vi "newTest.vi"(8 "error in (no error)":errorcluster, 11 "Data in":T1={"Report.lvclass"=refnum, "Norm"="", "last State"=enum."Initialize", "Norm ID"=0, "parameter"=[], "EMTestCWS500N.lvclass"=refnum, "CEG4500.lvclass"=refnum, "Tektronix RSA5106A.lvclass"=refnum, "erfolgreich"=FALSE, "log"="", "Kommentar"="", "Device Enum"=enum."emTestCWS500N", "Test Enum"=enum."HF-Felder", "debug"=FALSE, "tab"=enum."Hauptmenü", "ESD Pistol.lvclass"=refnum, "SubPnl Refnum"=refnum, "TabCtl Refnum"=refnum, "ButtonsEinblenden?"=FALSE}) -> (0 "error out":errorcluster, 2 "abbrechen":bool, 3 "Test out":refnum<class "Test.lvclass">)   [LabVIEW 2013]
uses:
  Main/controls/Data.ctl
  classes/Datastructure/Report/Report.lvclass
  classes/Devices/emTestCWS500N/EMTestCWS500N.lvclass
  classes/Devices/CEG4500/CEG4500.lvclass
  classes/Devices/Tektronix RSA5106A/Tektronix RSA5106A.lvclass
  ESD Pistol.lvclass
  Main/controls/State.ctl
  classes/Devices/DeviceInterface/Devices.ctl
  classes/Tests/TestInterface/Tests.ctl
  Tabs.ctl
  classes/Datastructure/Test/Test.lvclass
  classes/Datastructure/Norm/Norm.lvclass
  classes/Datastructure/Image/img.lvclass
panel:
  in  "Cancel Button":bool
  in  "Tree 2":string(tree)
  out "Norm":string caption="Test"
  in  "OK Button":bool
  in  "Add picture":bool
  in  "Kommentar":string
  in  "Test Name":string
  in  "Parameter":string[][](table)
  in  "number of pictures":i32
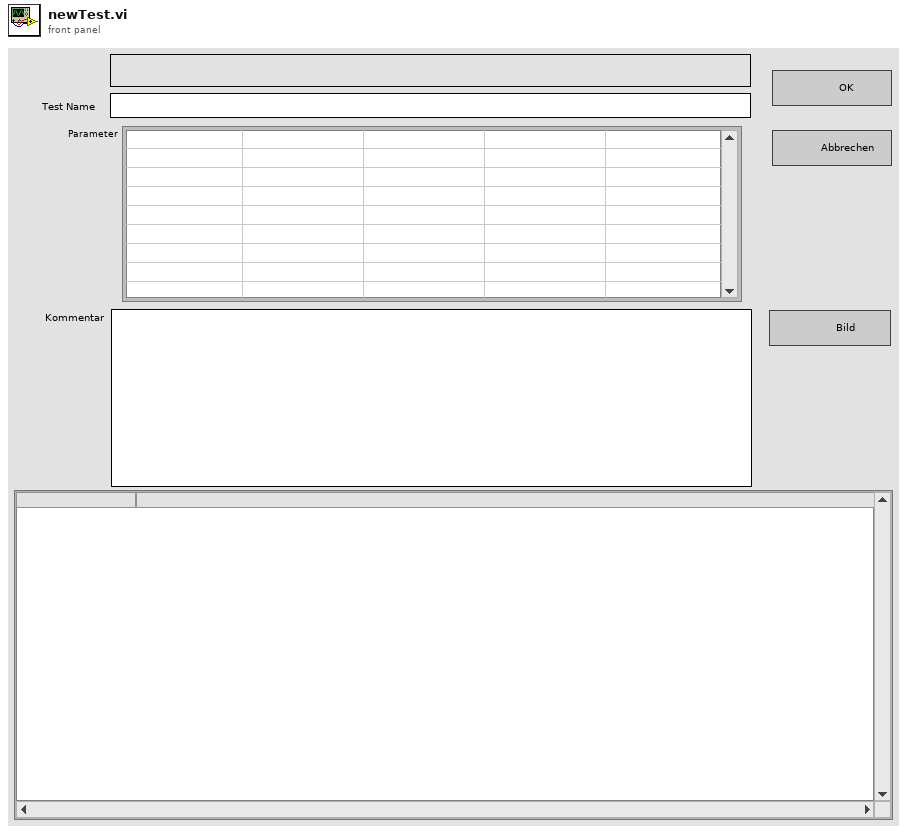
[diagram p1: front panel]
types:
  T1 = typedef "Data.ctl" = cluster{"Report.lvclass":refnum<class "Report.lvclass">, "Norm":string, "last State":T2, "Norm ID":i32, "parameter":string[][], "EMTestCWS500N.lvclass":refnum<class "EMTestCWS500N.lvclass">, "CEG4500.lvclass":refnum<class "CEG4500.lvclass">, "Tektronix RSA5106A.lvclass":refnum<class "Tektronix RSA5106A.lvclass">, "erfolgreich":bool, "log":string, "Kommentar":string, "Device Enum":T3, "Test Enum":T4, "debug":bool, "tab":T5, "ESD Pistol.lvclass":refnum<class "ESD Pistol.lvclass">, "SubPnl Refnum":refnum<vi>, "TabCtl Refnum":refnum<vi>, "ButtonsEinblenden?":bool}
  T2 = typedef "State.ctl" = enum16{"create Pdf", "load Report", "save Report", "do Test", "CDN Kalibrierung", "enter Report Parameters", "new Test", "Protokoll", "read Tree", "update Tree", "Fehler", "Initialize", "Wait for Event", "Exit"}
  T3 = typedef "Devices.ctl" = enum16{"unbekannt", "ESD Pistol", "Tektronix RSA5106A", "emTestCWS500N", "CEG-4500"}
  T4 = typedef "Tests.ctl" = enum16{"unbekannt", "Störaussendung", "Burst", "ESD", "Surge", "Spannungseinbruch", "HF-Felder"}
  T5 = typedef "Tabs.ctl" = enum32{"Hauptmenü", "Prüfbericht", "Einstellungen"}
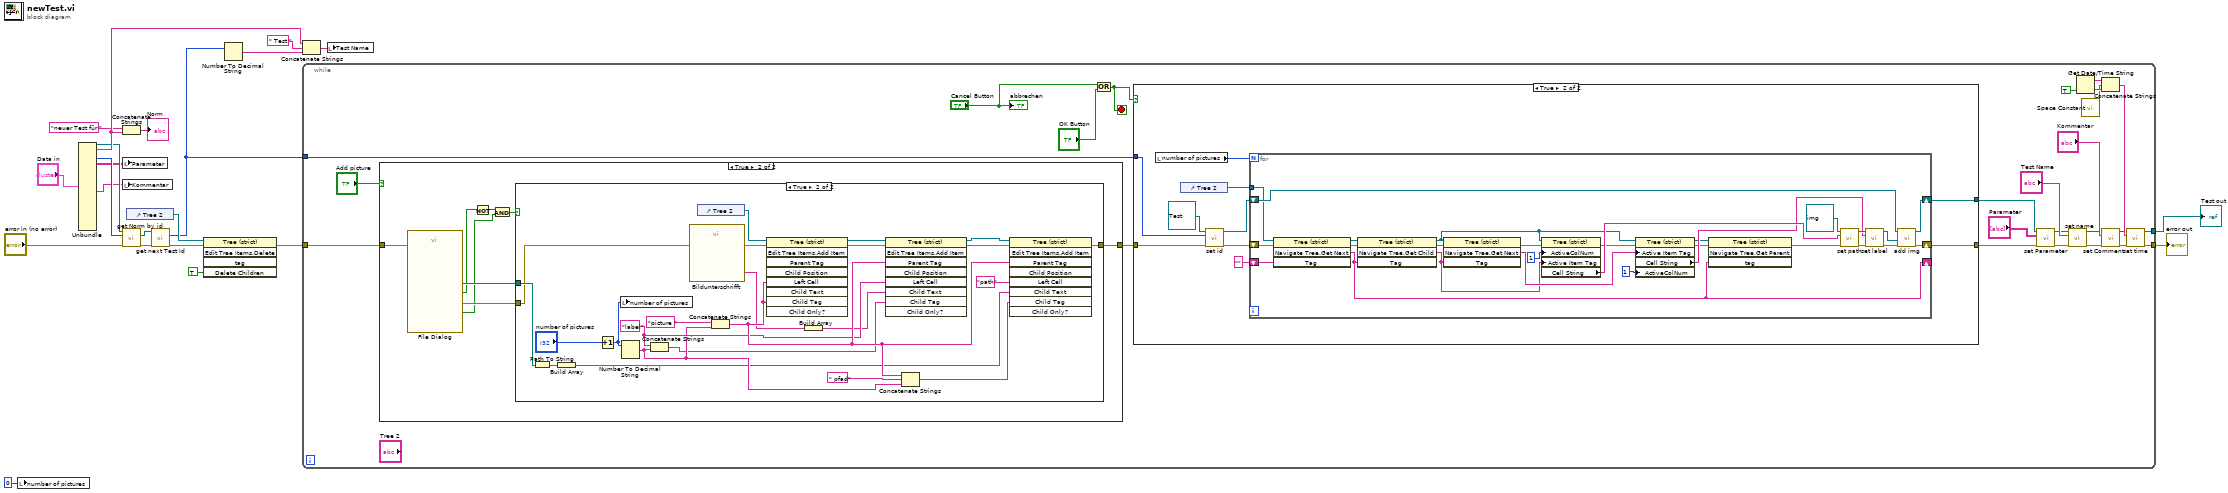
[diagram p0: block diagram]
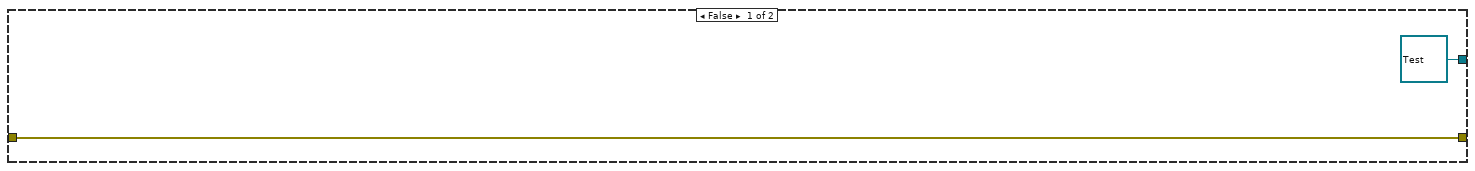
[diagram p2: hidden frame]
diagram:
  n1 = local write "number of pictures"(0 ("number of pictures")) -> ()
  n2 = Unbundle("Data in") -> ("Report.lvclass"=w19:refnum<class "Report.lvclass">, "Norm"=w21:string, "Norm ID"=w20:i32, "parameter"=w6:string[][], "Kommentar"=w10:string)  [unwired: 14 out]
  n3 = Concatenate Strings("neuer Test für ", w21) -> (→"Norm":string)
  n4 = local write "Parameter"(w6) -> ()
  n5 = local write "Kommentar"(w10) -> ()
  n6 = call-dynamic "get Norm by id.vi"("error in (no error)"="error in (no error)", "id"=w20, "Report (Eingang)"=w19) -> ("error out"=w4:errorcluster, "Norm.lvclass"=w5:refnum<class "Norm.lvclass">)  [unwired: 4 in, 3 out]
  n7 = control-ref of="Tree 2"() -> (w12:refnum<vi>)
  n8 = call-dynamic "get next Test Id.vi"("error in (no error)"=w4, "Norm in"=w5) -> ("error out"=w3:errorcluster, "id"=w2:u32)  [unwired: 7 in, 1 out]
  n9 = invoke class="Tree (strict)" method="Edit Tree Items.Delete"(reference=w12, error in=w3, "Delete Children"=TRUE ("Unterobjekte löschen?")) -> (error out=w13:errorcluster)  [unwired: 2 in, 4 out]
  n10 = Number To Decimal String(number=w2) -> (decimal integer string=w16:string)  [unwired: 1 in]
  n11 = Concatenate Strings(w21, " Test ", w16) -> (w8:string)
  n12 = while {
    tunnel: w13 -> [w45]
    tunnel: [w33] -> w15
    tunnel: [w32] -> w14
    tunnel: w2 -> [w23]
    stop <- w25 stop-if-true
    n13 = case shown="True" "Add picture" {
      tunnel: [w87 w93] -> w46
      tunnel: w45 -> [w87 w92]
      frame False {
      }
      frame True {
        n14 = call "File Dialog"("error in"=w92) -> ("selected path"=w95:path, "exists"=w88:bool, "cancelled"=w91:bool, "error out"=w94:errorcluster)  [unwired: 11 in]
        n15 = Not(x=w91) -> (.not. x?=w89:bool)
        n16 = And(x=w89, y=w88) -> (x .and. y?=w90:bool)
        n17 = case shown="True" w90 {
          tunnel: w95 -> [_ w110]
          tunnel: w94 -> [w96 w105]
          tunnel: [w96 w97] -> w93
          frame False {
          }
          frame True {
            w113 = "label" ("Left Cell String")
            n18 = Path To String(path=w110) -> (string=w106:string)
            n19 = Build Array(w106) -> (w109:string[])
            n20 = Increment(x="number of pictures") -> (x+1=w101:i32)
            n21 = local write "number of pictures"(w101) -> ()
            n22 = Number To Decimal String(number=w101) -> (decimal integer string=w112:string)  [unwired: 1 in]
            n23 = Concatenate Strings(w113, w112) -> (w111:string)
            n24 = call "Bildunterschrifft"("error in (no error)"=w105) -> ("Bildunterschrifft"=w104:string, "error out"=w100:errorcluster)  [unwired: 16 in, 1 out]
            n25 = control-ref of="Tree 2"() -> (w119:refnum<vi>)
            n26 = Concatenate Strings("picture " ("Left Cell String"), w112) -> (w114:string)
            n27 = invoke class="Tree (strict)" method="Edit Tree Items.Add Item"(reference=w119, error in=w100, "Left Cell"=w114, "Child Tag"=w114) -> (reference out=w108:refnum<vi>, error out=w99:errorcluster)  [unwired: 5 in, 7 out]
            n28 = Build Array(w104) -> (w103:string[])
            n29 = invoke class="Tree (strict)" method="Edit Tree Items.Add Item"(reference=w108, error in=w99, "Parent Tag"=w114, "Left Cell"=w113, "Child Text"=w103, "Child Tag"=w111) -> (reference out=w107:refnum<vi>, error out=w98:errorcluster)  [unwired: 3 in, 7 out]
            n30 = Concatenate Strings(w114, " pfad", w112) -> (w116:string)
            n31 = invoke class="Tree (strict)" method="Edit Tree Items.Add Item"(reference=w107, error in=w98, "Parent Tag"=w114, "Left Cell"="path" ("Left Cell String"), "Child Text"=w109, "Child Tag"=w116) -> (error out=w97:errorcluster)  [unwired: 3 in, 8 out]
          }
        }
      }
    }
    n32 = Or(x="Cancel Button", y="OK Button") -> (x .or. y?=w25:bool)
    n33 = case shown="True" w25 {
      tunnel: [refnum<class "Test.lvclass"> refnum ("Segment.lvclass") w59] -> w31
      tunnel: [w48 w58] -> w30
      tunnel: w46 -> [w48 w52]
      tunnel: w23 -> [_ w53]
      frame False {
      }
      frame True {
        n34 = local read "number of pictures"() -> (w56:i32)
        n35 = control-ref of="Tree 2"() -> (w57:refnum<vi>)
        n36 = call-dynamic "set id.vi"("error in (no error)"=w52, "id"=w53, "Test in"=refnum<class "Test.lvclass"> refnum ("Segment.lvclass")) -> ("error out"=w51:errorcluster, "Test out"=w50:refnum<class "Test.lvclass">)  [unwired: 7 in]
        n37 = for {
          N: w56 -> [_]
          tunnel: w57 -> [w65]
          shift-right: [w77] -> w59
          shift-left: w50 -> [w85]
          shift-right: [w70] -> w58
          shift-left: w51 -> [w69]
          shift-right: [w64] -> _
          shift-left: "" ("Navigate Tree:Get Next Item") -> [w63]
          n38 = invoke class="Tree (strict)" method="Navigate Tree.Get Next"(reference=w65, error in=w69, "Tag"=w63) -> (reference out=w86:refnum<vi>, error out=w76:errorcluster, "Navigate Tree:Get Next Item"=w64:string)  [unwired: 1 in, 1 out]
          n39 = invoke class="Tree (strict)" method="Navigate Tree.Get Child"(reference=w86, error in=w76, "Tag"=w64) -> (reference out=w81:refnum<vi>, error out=w75:errorcluster, "Navigate Tree:Get Child"=w62:string)  [unwired: 1 in, 1 out]
          n40 = invoke class="Tree (strict)" method="Navigate Tree.Get Next"(reference=w81, error in=w75, "Tag"=w62) -> (error out=w74:errorcluster, "Navigate Tree:Get Next Item"=w80:string)  [unwired: 1 in, 2 out]
          n41 = property class="Tree (strict)"(reference=w81, error in=w74, "ActiveColNum"=1 ("Active Cell:Active Column Number"), "Active Item Tag"=w62) -> (error out=w73:errorcluster, "Cell String"=w82:string)  [unwired: 1 out]
          n42 = property class="Tree (strict)"(reference=w81, error in=w73, "Active Item Tag"=w80, "ActiveColNum"=1 ("Active Cell:Active Column Number")) -> (reference out=w66:refnum<vi>, error out=w61:errorcluster, "Cell String"=w79:string)
          n43 = invoke class="Tree (strict)" method="Navigate Tree.Get Parent"(reference=w66, error in=w61, "tag"=w64) -> (error out=w60:errorcluster)  [unwired: 1 in, 3 out]
          n44 = call-dynamic "set path.vi"("error in (no error)"=w60, "path"=w82, "img (Eingang)"=refnum<class "img.lvclass"> refnum ("img.lvclass")) -> ("error out"=w72:errorcluster, "img (Ausgang)"=w84:refnum<class "img.lvclass">)  [unwired: 7 in]
          n45 = call-dynamic "set label.vi"("error in (no error)"=w72, "label"=w79, "img (Eingang)"=w84) -> ("error out"=w71:errorcluster, "img (Ausgang)"=w78:refnum<class "img.lvclass">)  [unwired: 7 in]
          n46 = call-dynamic "add img.vi"("error in (no error)"=w71, "img.lvclass"=w78, "Test (Eingang)"=w85) -> ("error out"=w70:errorcluster, "Test (Ausgang)"=w77:refnum<class "Test.lvclass">)  [unwired: 6 in]
        }
      }
    }
    n47 = call-dynamic "set Parameter.vi"("error in (no error)"=w30, "Parameter"="Parameter", "Test (Eingang)"=w31) -> ("error out"=w27:errorcluster, "Test (Ausgang)"=w28:refnum<class "Test.lvclass">)  [unwired: 7 in]
    n48 = call-dynamic "set name.vi"("error in (no error)"=w27, "name"="Test Name", "Test (Eingang)"=w28) -> ("error out"=w34:errorcluster, "Test (Ausgang)"=w37:refnum<class "Test.lvclass">)  [unwired: 7 in]
    n49 = Get Date/Time String(want seconds? (F)=TRUE) -> (date string=w41:string, time string=w42:string)  [unwired: 2 out]
    n50 = call <vilib>:"Space Constant.vi"() -> ("String"=w40:string)
    n51 = Concatenate Strings(w41, w40, w42) -> (w38:string)
    n52 = call-dynamic "set Comment.vi"("error in (no error)"=w34, "Comment"="Kommentar", "Test (Eingang)"=w37) -> ("error out"=w35:errorcluster, "Test (Ausgang)"=w36:refnum<class "Test.lvclass">)  [unwired: 7 in]
    n53 = call-dynamic "set time.vi"("error in (no error)"=w35, "time"=w38, "Test (Eingang)"=w36) -> ("error out"=w33:errorcluster, "Test (Ausgang)"=w32:refnum<class "Test.lvclass">)  [unwired: 7 in]
    "abbrechen" <- "Cancel Button"
  }
  "error out" <- w15
  "Test out" <- w14
  n54 = local write "Test Name"(w8) -> ()
